vi "Key Value Lookup FGV.vi"(7 "Method (Get)":enum16{"Get", "Set"}(ring), 8 "error in (no error)":errorcluster, 10 "Value In":variant, 11 "Key":string) -> (0 "error out":errorcluster, 3 "Value Out":variant)   [LabVIEW 2019]
doc: "This is a simple use case for a varient. It is similar to the FGV. The difference is that the data is stored in a variant attribute rather than a shift register. The architect may want to compare the two techniques for performance. This also illustrates that several design patterns can be used for the same use case.\n\nAAL 9/09"
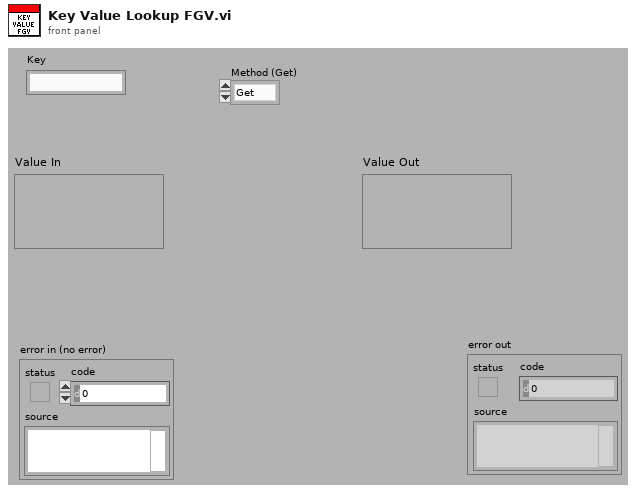
[diagram p1: front panel]
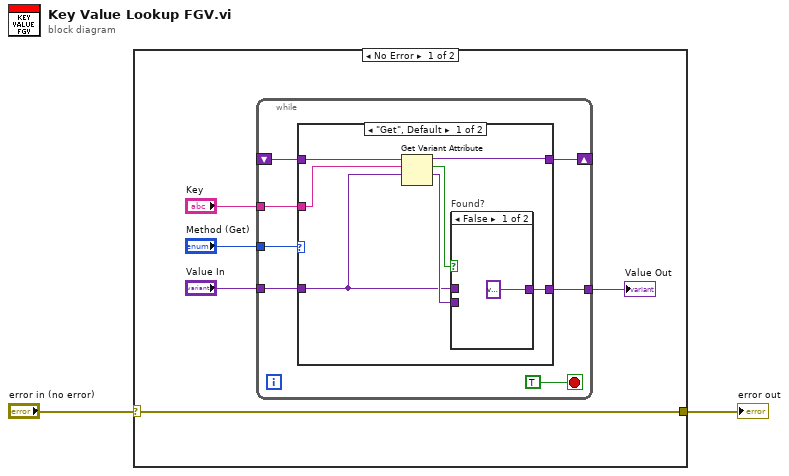
[diagram p0: block diagram]
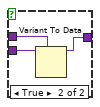
[diagram p2: hidden frame]
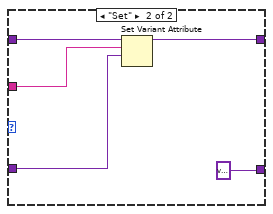
[diagram p3: hidden frame]
diagram:
  n1 = case shown="No Error" "error in (no error)" {
    selector: "error in (no error)" -> [w7 w31]
    tunnel: [w7 w31] -> w1
    frame No Error {
      n2 = while {
        tunnel: "Method (Get)" -> [w14]
        tunnel: "Value In" -> [w13]
        tunnel: "Key" -> [w10]
        tunnel: [w9] -> w3
        shift-right: [w11] -> _
        shift-left: _ -> [w12]
        stop <- TRUE stop-if-true
        n3 = case shown="\"Get\", Default" w14 {
          tunnel: w13 -> [w16 w27]
          tunnel: w12 -> [w21 w30]
          tunnel: [w20 w29] -> w11
          tunnel: w10 -> [w19 w28]
          tunnel: [w17 variant ("Data Out")] -> w9
          frame "Get", Default {
            n4 = Get Variant Attribute(Variant=w21, name=w19, default value (empty Variant)=w16) -> (duplicate Variant=w20:variant, found=w15:bool, value=w18:variant)  [unwired: 1 in, 1 out]
            n5 = case "Found?" shown="False" w15 {
              tunnel: w18 -> [_ w25]
              tunnel: [variant ("Set Function") w24] -> w17
              tunnel: w16 -> [_ w23]
              frame False {
              }
              frame True {
                n6 = Variant To Data(type=w23, Variant=w25) -> (data=w24:variant)  [unwired: 1 in, 1 out]
              }
            }
          }
          frame "Set" {
            n7 = Set Variant Attribute(Variant=w30, name=w28, value=w27) -> (Variant out=w29:variant)  [unwired: 1 in, 2 out]
          }
        }
      }
      "Value Out" <- w3
    }
    frame Error {
    }
  }
  "error out" <- w1
